vi "测试.vi"() -> ()   [LabVIEW 2019]
panel:
  out "time":cluster{"计时？":bool, "计时 (ms)":u32}
  in  "结束":bool
  in  "重置":bool
  in  "停止":bool
  in  "开始":bool
  in  "Timer.lvclass":refnum<class "Timer.lvclass">
  out "statue":T1
  out "Login":T2
  in  "User Management Model.lvclass":refnum<class "User Management Model.lvclass">
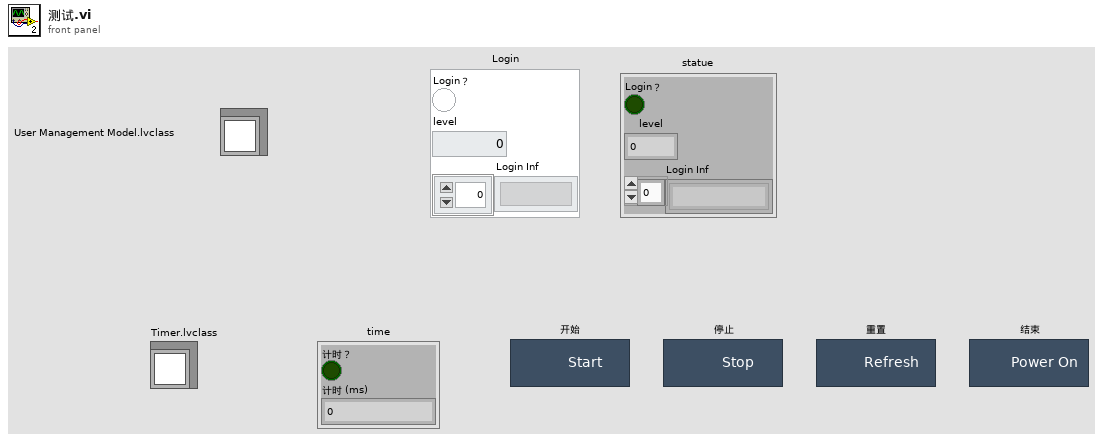
[diagram p1: front panel]
types:
  T1 = typedef "User Management Model.lvclass/ObjectAttributes.ctl" = cluster{"Login？":bool, "level":i32, "Login Inf":string[]}
  T2 = cluster{"Login？":bool, "level":dbl, "Login Inf":string[]}
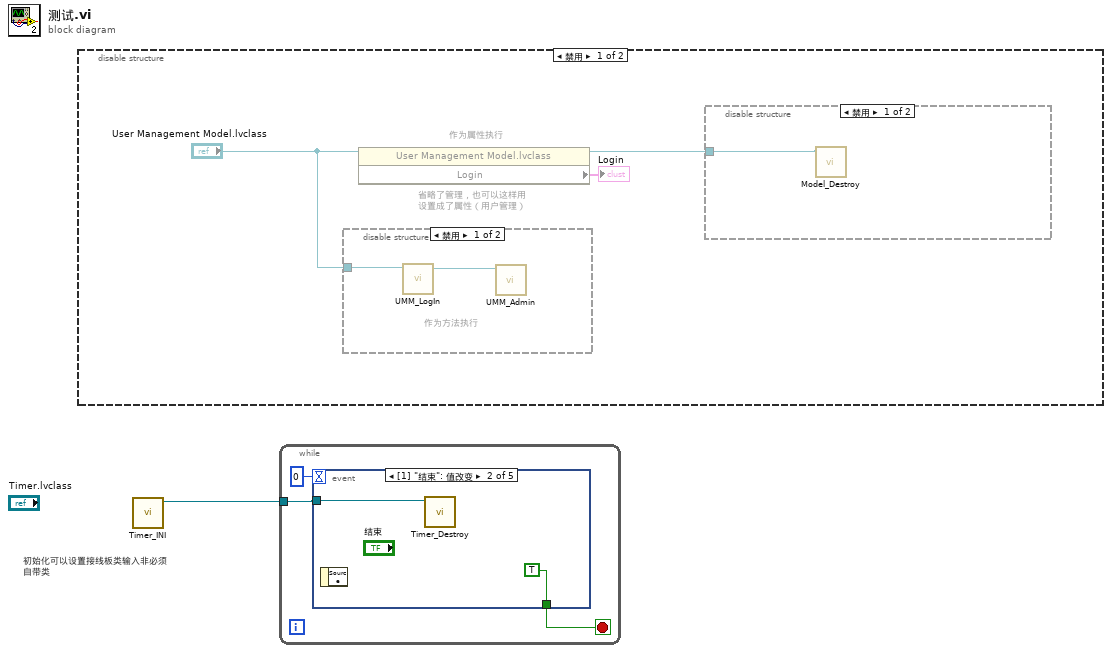
[diagram p0: block diagram]
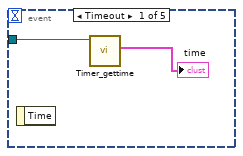
[diagram p2: hidden frame]
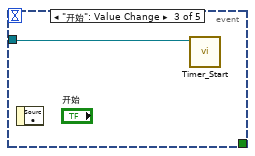
[diagram p3: hidden frame]
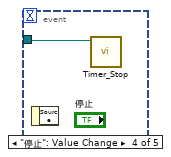
[diagram p4: hidden frame]
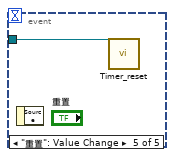
[diagram p5: hidden frame]
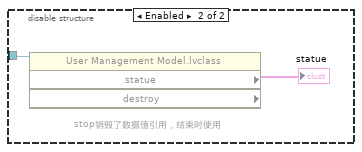
[diagram p6: hidden frame]
diagram:
  # "初始化可以设置接线板类输入非必须\n自带类"
  n1 = disable-structure shown="禁用" {
    frame Disabled {
      # "省略了管理，也可以这样用\n设置成了属性（用户管理）"
      # "作为属性执行"
      n2 = disable-structure shown="禁用" {
        disable-tunnel: "User Management Model.lvclass" -> [w9 _]
        frame Disabled {
          # "作为方法执行"
          n3 = call-dynamic "UMM_LogIn.vi"("User Management Model 输入"=w9) -> ("User Management Model 输出"=w8:refnum<class "User Management Model.lvclass">)  [unwired: 8 in, 2 out]
          n4 = call-dynamic "UMM_Admin.vi"("User Management Model 输入"=w8) -> ()  [unwired: 8 in, 3 out]
        }
        frame Enabled {
        }
      }
      n5 = property class="User Management Model.lvclass"(reference="User Management Model.lvclass") -> (reference out=w2:refnum<class "User Management Model.lvclass">, "Login"=→"Login":T1)  [unwired: 1 in, 1 out]
      n6 = disable-structure shown="禁用" {
        disable-tunnel: w2 -> [w5 w7]
        frame Disabled {
          n7 = call "Model_Destroy.vi"("User Management Model 输入"=w5) -> ()  [unwired: 8 in, 3 out]
        }
        frame Enabled {
          # "stop销毁了数据值引用，结束时使用"
          n8 = property class="User Management Model.lvclass" props=["statue", "destroy"](reference=w7) -> ("statue"=→"statue":T1)  [unwired: 1 in, 3 out]
        }
      }
    }
    frame Enabled {
    }
  }
  n9 = call "Timer_INI.vi"() -> ("Timer 输出"=w1:refnum<class "Timer.lvclass">)  [unwired: 10 in, 1 out]
  n10 = while {
    tunnel: w1 -> [w10]
    stop <- w12 stop-if-true
    n11 = event shown="[1] \"结束\": 值改变" {
      selector: _ -> [_ _ _ _ _]
      dyn-events: _ -> [_ _ _ _ _]
      timeout: 0 -> [_ _ _ _ _]
      tunnel: w10 -> [w14 w15 w17 w18 w19]
      tunnel: [_ TRUE ("结束") _ _ _] -> w12
      event Timeout {
        n12 = event-data() -> ()  [unwired: 1 in, 1 out]
        n13 = call "Timer_gettime.vi"("Timer 输入"=w14) -> ("time"=→"time":cluster{"计时？":bool, "计时 (ms)":u32})  [unwired: 8 in, 2 out]
      }
      event "结束": Value Change {
        n14 = event-data() -> ()  [unwired: 1 in, 1 out]
        n15 = call "Timer_Destroy.vi"("Timer 输入"=w15) -> ()  [unwired: 9 in, 2 out]
      }
      event "开始": Value Change {
        n16 = event-data() -> ()  [unwired: 1 in, 1 out]
        n17 = call "Timer_Start.vi"("Timer 输入"=w17) -> ()  [unwired: 9 in, 2 out]
      }
      event "停止": Value Change {
        n18 = event-data() -> ()  [unwired: 1 in, 1 out]
        n19 = call "Timer_Stop.vi"("Timer 输入"=w18) -> ()  [unwired: 9 in, 2 out]
      }
      event "重置": Value Change {
        n20 = event-data() -> ()  [unwired: 1 in, 1 out]
        n21 = call "Timer_reset.vi"("Timer 输入"=w19) -> ()  [unwired: 9 in, 2 out]
      }
    }
  }
